vi "Intake_Ball_Globals.vi"() -> ()   [LabVIEW 2018]
uses:
  Subsytems/Intake_Ball/Intake_Ball_Notifier.ctl
  Subsytems/Intake_Ball/Intake_Ball_Control_Type.ctl
panel:
  in  "Intake_Ball_Set_Ref":refnum<notifier>
  in  "Intake_Ball_Execute_Ref":refnum<notifier>
  in  "Intake_Ball_Execute_Notifier":string="Intake_Ball_Execute_Notifier"
  in  "Intake_Ball_Set_Notifier":string="Intake_Ball_Set_Notifier"
  in  "Intake_Ball_Motor":string="Intake_Ball_Motor"
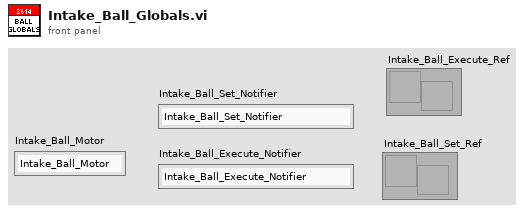
[diagram p1: front panel]
diagram:
